vi "Write Vehicle Location.vi"(8 "error in (no error)":errorcluster, 10 "Vehicle Location":cluster{"x":dbl, "y":dbl}, 11 "Simulator in":refnum<class "Simulator.lvclass">) -> (0 "error out":errorcluster, 3 "Simulator out":refnum<class "Simulator.lvclass">)   [LabVIEW 2011, in "Simulator.lvclass"]
uses:
  Simulator.lvclass
  Simulator.lvclass/Simulator.ctl
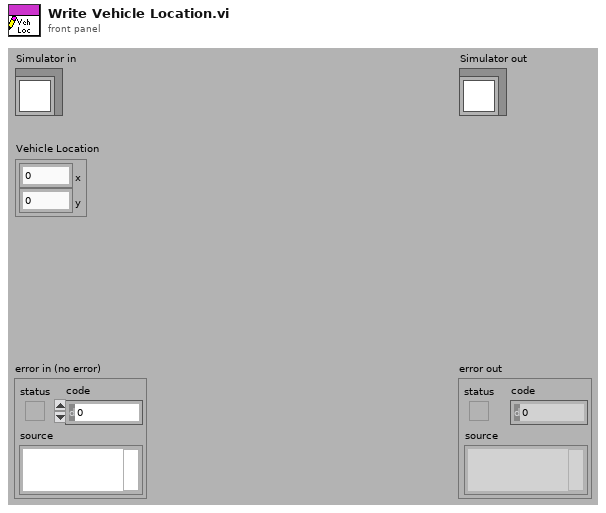
[diagram p1: front panel]
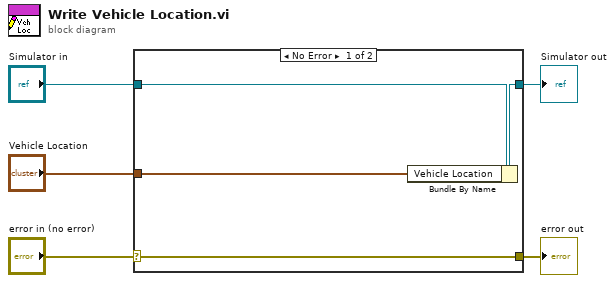
[diagram p0: block diagram]
diagram:
  n1 = case shown="No Error" "error in (no error)" {
    selector: "error in (no error)" -> [w9 w10]
    tunnel: [w9 w10] -> w4
    tunnel: [w7 w11] -> w2
    tunnel: "Simulator in" -> [w8 w11]
    tunnel: "Vehicle Location" -> [w6 _]
    frame No Error {
      n2 = Bundle By Name(cluster=w8, "Vehicle Location"=w6) -> (w7:refnum<class "Simulator.lvclass">)
    }
    frame Error {
    }
  }
  "error out" <- w4
  "Simulator out" <- w2
